vi "Read To End.vi"(8 "error in (no error)":errorcluster, 10 "Stream Reader Ref":refnum<k24>, 11 "Shell Stream Reference":refnum<k24>) -> (0 "error out":errorcluster, 1 "DataAvailable":bool, 2 "ReadToEnd":string)   [LabVIEW 2017, in "SSH.lvlib"]
doc: "Reads the data currently in the StreamReader buffer - indicates if there is any data available or if the string will be empty"
uses:
  SSH.lvlib
  C:/Users/ukhornp/Documents/SSH/References/Renci.SshNet.dll
  References/Renci.SshNet.dll
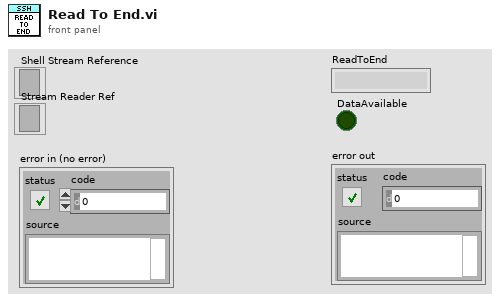
[diagram p1: front panel]
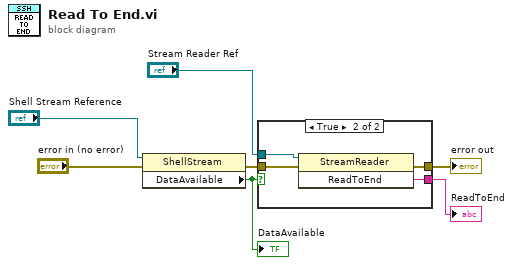
[diagram p0: block diagram]
diagram:
  n1 = property class="ShellStream"(reference="Shell Stream Reference", error in="error in (no error)") -> (error out=w6:errorcluster, "DataAvailable"=w7:bool)  [unwired: 1 out]
  "DataAvailable" <- w7
  n2 = case shown="True" w7 {
    tunnel: w6 -> [w8 w12]
    tunnel: [w8 w11] -> w4
    tunnel: [_ w10] -> w3
    tunnel: "Stream Reader Ref" -> [_ w9]
    frame False {
    }
    frame True {
      n3 = invoke class="StreamReader" method="ReadToEnd"(reference=w9, error in=w12) -> (error out=w11:errorcluster, "ReadToEnd"=w10:string)  [unwired: 1 in, 1 out]
    }
  }
  "error out" <- w4
  "ReadToEnd" <- w3
